vi "CreatorComplete.vi"(8 "error in (no error)":errorcluster, 11 "QControlWizard in":refnum<class "QControl Creation Wizard.lvclass">) -> (0 "error out":errorcluster, 3 "QControlWizard (dup)":refnum<class "QControl Creation Wizard.lvclass">)   [LabVIEW 2015, in "QControl Creation Wizard.lvclass"]
doc: "<b> </b> <b> </b>\n©2016 Q Software Innovations, LLC (QSI)\nwritten by Quentin Alldredge\nproduced in LabVIEW 2015\n\nsupport@qsoftwareinnovations.com\nwww.qsoftwareinnovations.com\n\nAll rights reserved.\n\nRedistribution and use in source and binary forms, with or without modification, are permitted provided that the following conditions are met:\n\n * Redistributions of source code must retain the above copyright notice, this list of conditions and the following disclaimer.\n * Redistributions in binary form must reproduce the above copyright notice, this list of conditions and the following disclaimer in the documentation and/or other materials provided with the distribution.\n * Neither the name of Q Software Innovations, LLC. nor the names of its contributors may be used to endorse or promote products derived from this software without specific prior written permission.\n\nTHIS SOFTWARE IS PROVIDED BY THE COPYRIGHT HOLDERS AND CONTRIBUTORS \"AS IS\" AND ANY EXPRESS OR IMPLIED WARRANTIES, INCLUDING, BUT NOT LIMITED TO, THE IMPLIED WARRANTIES OF MERCHANTABILITY AND FITNESS FOR A PARTICULAR PURPOSE ARE DISCLAIMED. IN NO EVENT SHALL THE COPYRIGHT OWNER OR CONTRIBUTORS BE LIABLE FOR ANY DIRECT, INDIRECT, INCIDENTAL, SPECIAL, EXEMPLARY, OR CONSEQUENTIAL DAMAGES (INCLUDING, BUT NOT LIMITED TO, PROCUREMENT OF SUBSTITUTE GOODS OR SERVICES; LOSS OF USE, DATA, OR PROFITS; OR BUSINESS INTERRUPTION) HOWEVER CAUSED AND ON ANY THEORY OF LIABILITY, WHETHER IN CONTRACT, STRICT LIABILITY, OR TORT (INCLUDING NEGLIGENCE OR OTHERWISE) ARISING IN ANY WAY OUT OF THE USE OF THIS SOFTWARE, EVEN IF ADVISED OF THE POSSIBILITY OF SUCH DAMAGE."
uses:
  QControl Creation Wizard.lvclass
  QControl Creation Wizard.lvclass/QControl Creation Wizard.ctl
  QControl Classes/StatusHistory/Add Item.vi
  New QControl Info/New QControl Info.lvclass
  QControl Classes/StatusHistory/StatusHistory.lvclass
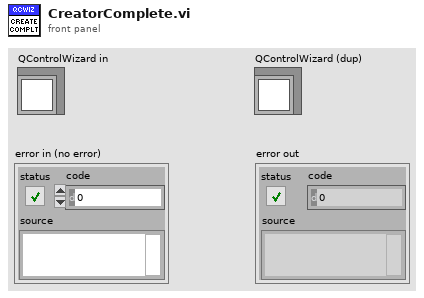
[diagram p1: front panel]
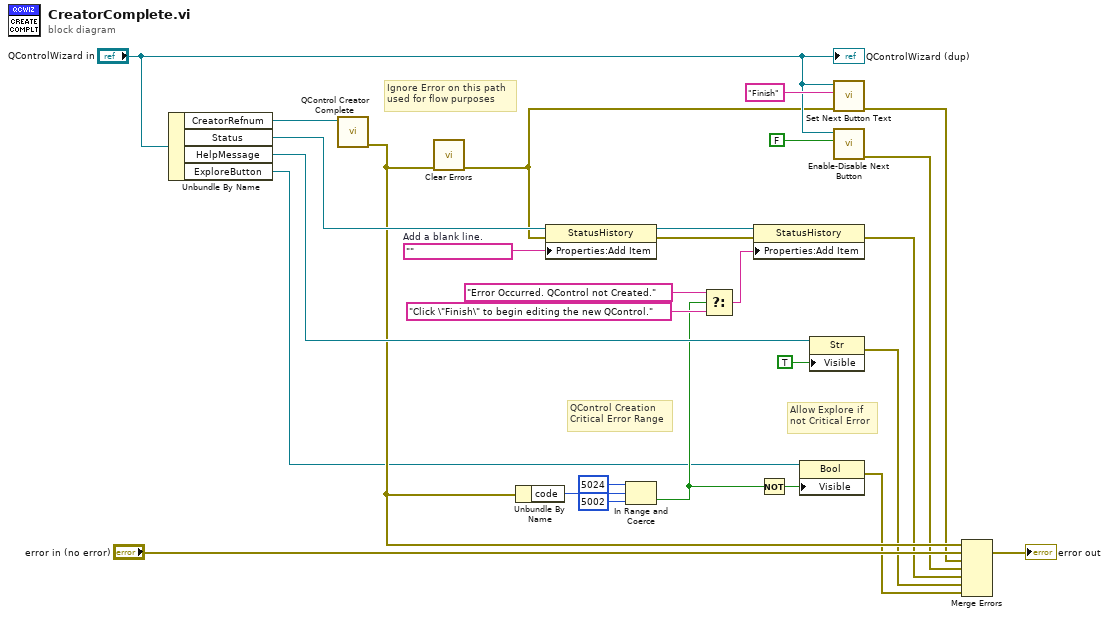
[diagram p0: block diagram]
diagram:
  w14 = ""  # Add a blank line.
  (unwired) 5021 ("upper limit")
  # "Ignore Error on this path\nused for flow purposes"
  # "Allow Explore if \nnot Critical Error"
  # "QControl Creation \nCritical Error Range"
  n1 = Unbundle By Name("QControlWizard in") -> ("CreatorRefnum"=w17:refnum<vi>, "Status"=w16:refnum<class "StatusHistory.lvclass">, "HelpMessage"=w13:refnum<vi>, "ExploreButton"=w8:refnum<vi>)
  n2 = call "QControl Creator Complete.vi"("CreatorRefnum"=w17) -> ("error out"=w9:errorcluster)  [unwired: 9 in]
  n3 = call <vilib>:"Clear Errors.vi"("error in (no error)"=w9) -> ("error out"=w1:errorcluster)  [unwired: 5 in, 1 out]
  n4 = Unbundle By Name(w9) -> ("code"=w25:i32)
  n5 = property class="StatusHistory"(reference=w16, error in=w1, "Properties:Add Item"=w14) -> (reference out=w15:refnum<class "StatusHistory.lvclass">, error out=w10:errorcluster)
  n6 = In Range and Coerce(upper limit=5024, x=w25, lower limit=5002 ("upper limit")) -> (In Range?=w12:bool)  [unwired: 1 out]
  n7 = Select(t="Error Occurred. QControl not Created." ("Add Item"), s=w12, f="Click \"Finish\" to begin editing the new QControl." ("Add Item")) -> (s? t:f=w20:string)
  n8 = property class="StatusHistory"(reference=w15, error in=w10, "Properties:Add Item"=w20) -> (error out=w4:errorcluster)  [unwired: 1 out]
  n9 = Not(x=w12) -> (.not. x?=w22:bool)
  n10 = property class="Bool"(reference=w8, "Visible"=w22) -> (error out=w2:errorcluster)  [unwired: 1 in, 1 out]
  n11 = property class="Str"(reference=w13, "Visible"=TRUE) -> (error out=w3:errorcluster)  [unwired: 1 in, 1 out]
  n12 = call "Set Next Button Text.vi"("error in (no error)"=w1, "Text"="Finish", "QControlWizard in"="QControlWizard in") -> ("error out"=w6:errorcluster)  [unwired: 7 in, 1 out]
  n13 = call "Enable-Disable Next Button.vi"("Disable Next Button?"=FALSE, "QControlWizard in"="QControlWizard in") -> ("error out"=w5:errorcluster)  [unwired: 8 in, 1 out]
  n14 = Merge Errors(w9, "error in (no error)", w6, w5, w4, w3, w2) -> (→"error out":errorcluster)
  "QControlWizard (dup)" <- "QControlWizard in"
